vi "String.LineFeed Delimited String to 1D Str Array.vi"(11 "String":string) -> (3 "Array":string[](array[string]))   [LabVIEW 2019]
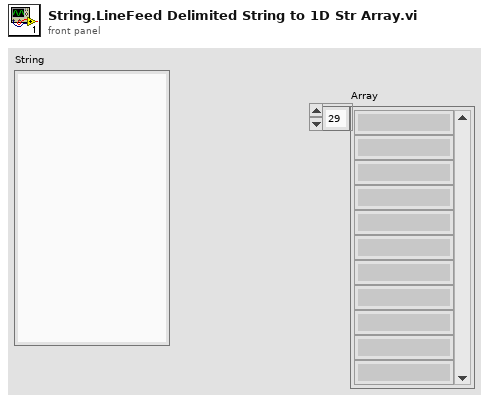
[diagram p1: front panel]
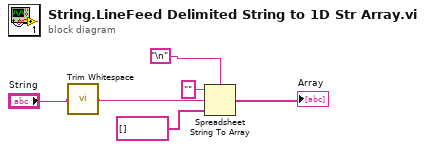
[diagram p0: block diagram]
diagram:
  n1 = call <vilib>:"Trim Whitespace.vi"("string"="String") -> ("trimmed string"=w1:string)  [unwired: 1 in]
  n2 = Spreadsheet String To Array(delimiter (Tab)="\n", format string="", spreadsheet string=w1, array type (2D Dbl)=string[] [] ("Array")) -> (array=→"Array":string[])
